vi "cut lf cr.vi"(11 "strin":string) -> (3 "strout":string)   [LabVIEW 2020]
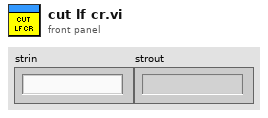
[diagram p1: front panel]
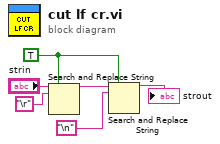
[diagram p0: block diagram]
diagram:
  w1 = TRUE ("tout remplacer ? (F)")
  n1 = Search and Replace String ("Rechercher et remplacer une chaîne")(replace all?=w1, input string="strin", search string="\r") -> (result string=w4:string)  [unwired: 5 in, 3 out]
  n2 = Search and Replace String ("Rechercher et remplacer une chaîne")(replace all?=w1, input string=w4, search string="\n") -> (result string=→"strout":string)  [unwired: 5 in, 3 out]
